vi "Calculate Vertex Array.vi"(8 "error in (no error)":errorcluster, 9 "Coordinates System":enum16{"Cartesian", "Cylindrical", "Spherical"}(ring)=enum."Spherical", 10 "3D Mesh Datatype.lvclass in":refnum<class "3D Ribbon Datatype.lvclass">, 11 "Plot Representation In":T1) -> (0 "error out":errorcluster, 1 "Dup Coordinates System":enum16{"Cartesian", "Cylindrical", "Spherical"}(ring)=enum."Spherical", 2 "3D Mesh Datatype.lvclass out":refnum<class "3D Ribbon Datatype.lvclass">, 3 "Plot Representation Out":T1)   [LabVIEW 2020, in "3D Ribbon Datatype.lvclass"]
uses:
  <vilib>/Math Plots/3D Math Plots/3D Ribbon/3D Ribbon Datatype/3D Ribbon Datatype.lvclass
  <vilib>/Math Plots/3D Math Plots/3D Plot/3D Plot/Typedef/Plot Representation.ctl
  <vilib>/Math Plots/3D Math Plots/3D Plot/3D Plot/Typedef/Range Clusters.ctl
  <vilib>/Math Plots/3D Math Plots/3D Plot/3D Plot/Typedef/Mesh Data.ctl
  <vilib>/Math Plots/3D Math Plots/3D Ribbon/3D Ribbon Datatype/3D Ribbon Datatype.lvclass/3D Ribbon Datatype.ctl
  <vilib>/Math Plots/3D Math Plots/3D Plot/3D Plot Datatype/3D Plot Datatype.lvclass
  <vilib>/Math Plots/3D Math Plots/3D Plot/3D Plot/3D Plot.lvclass
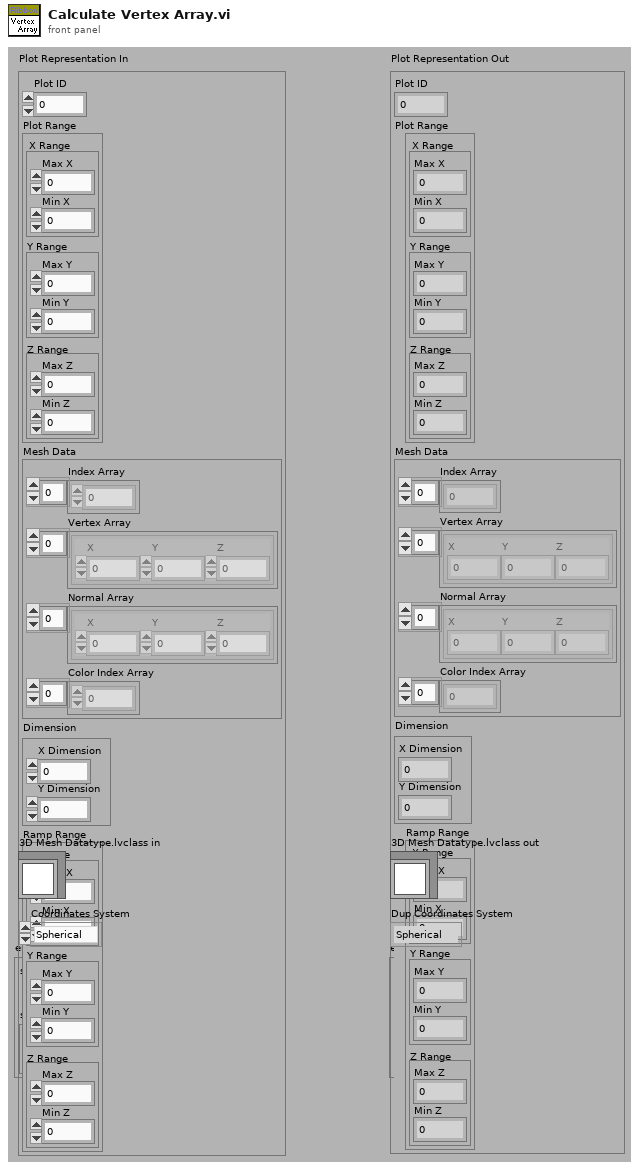
[diagram p1: front panel]
types:
  T1 = typedef "3D Plot.lvclass/Plot Representation.ctl" = cluster{"Plot ID":i32, "Plot Range":T2, "Mesh Data":T3, "Dimension":cluster{"X Dimension":i32, "Y Dimension":i32}, "Ramp Range":T2}
  T2 = typedef "3D Plot.lvclass/Range Clusters.ctl" = cluster{"X Range":cluster{"Max X":sgl, "Min X":sgl}, "Y Range":cluster{"Max Y":sgl, "Min Y":sgl}, "Z Range":cluster{"Max Z":sgl, "Min Z":sgl}}
  T3 = typedef "3D Plot.lvclass/Mesh Data.ctl" = cluster{"Index Array":u32[], "Vertex Array":cluster{"X":sgl, "Y":sgl, "Z":sgl}[], "Normal Array":cluster{"X":sgl, "Y":sgl, "Z":sgl}[], "Color Index Array":i32[]}
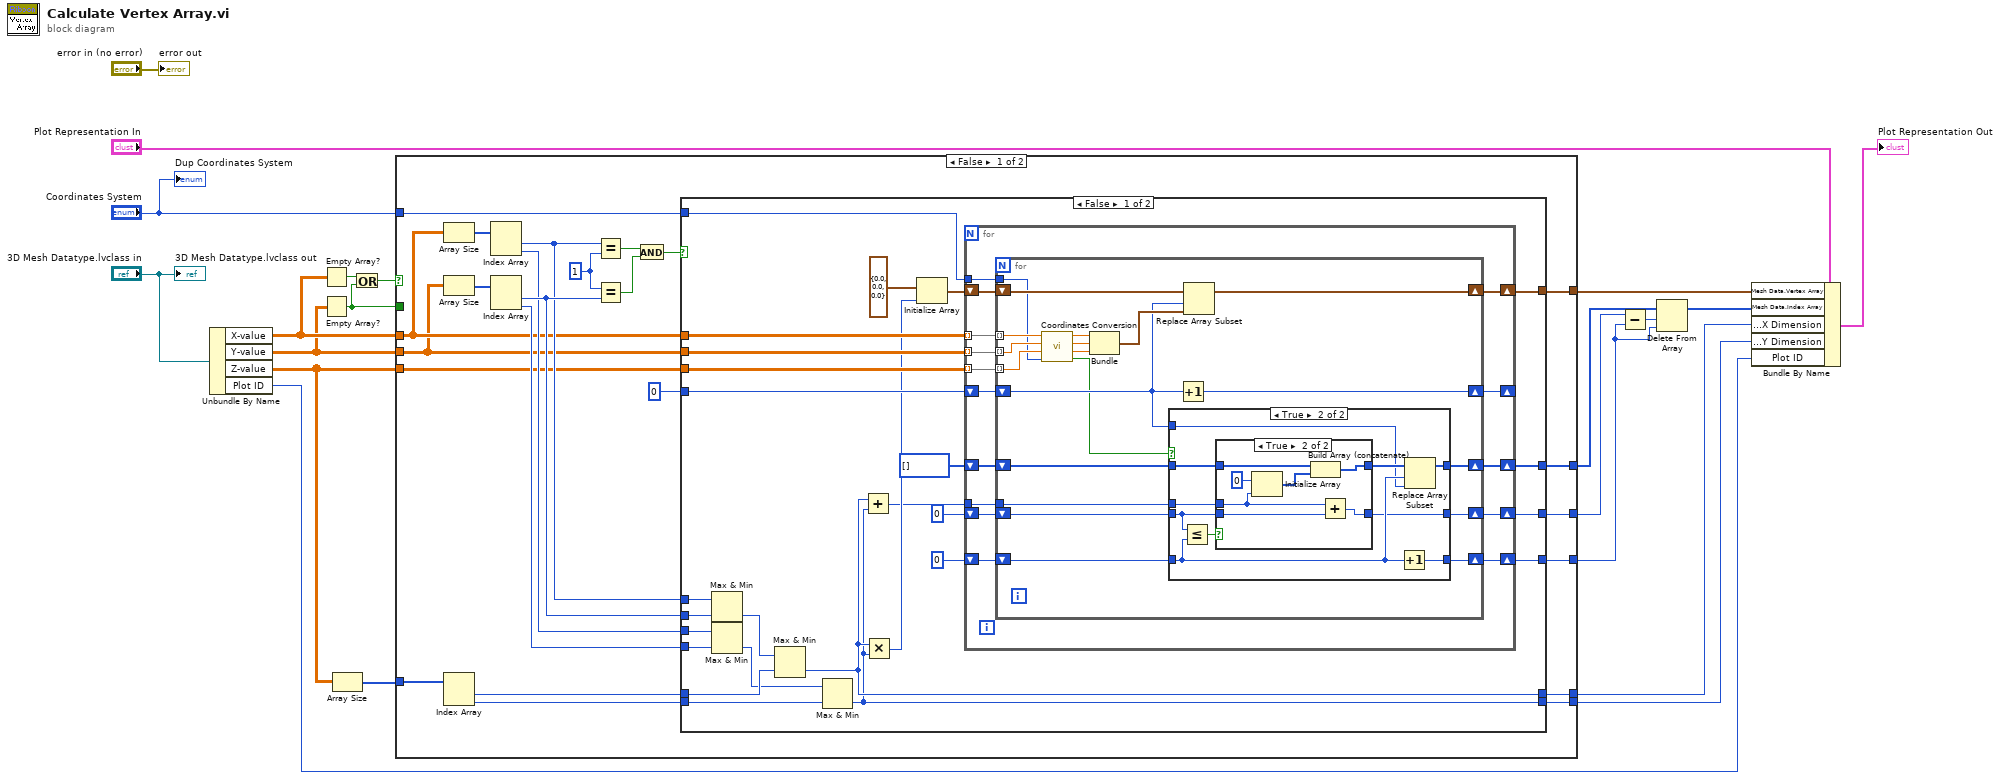
[diagram p0: block diagram]
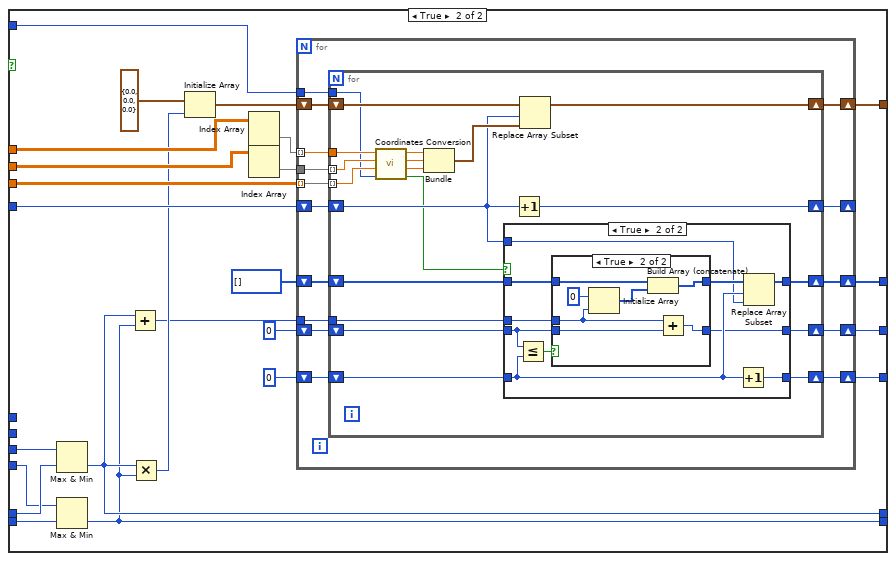
[diagram p4: hidden frame]
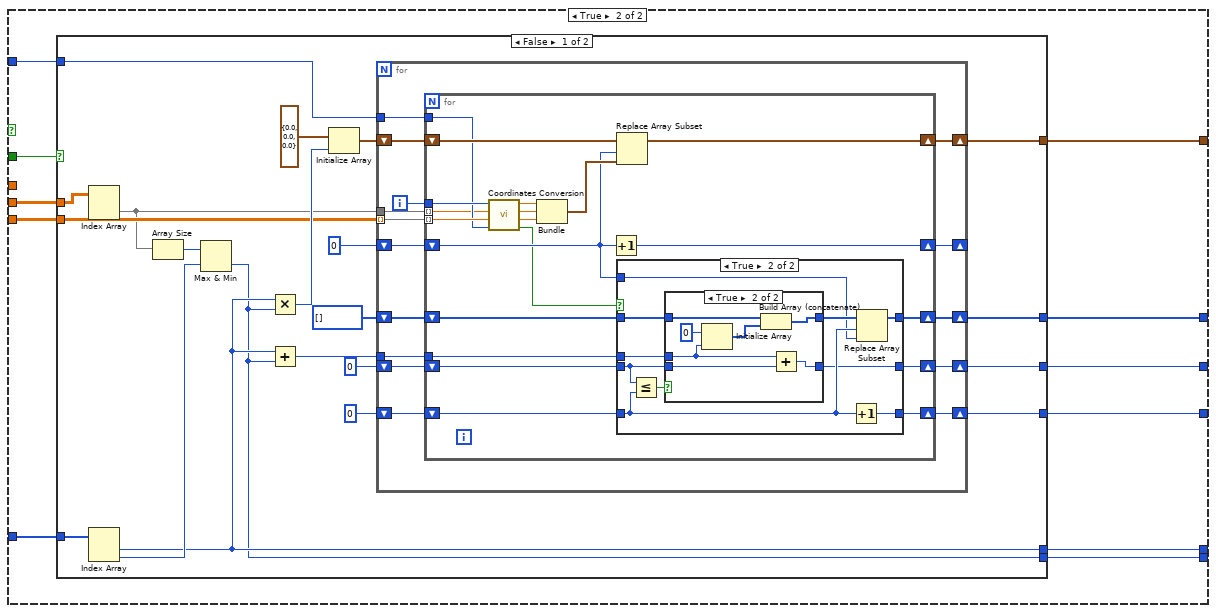
[diagram p7: hidden frame]
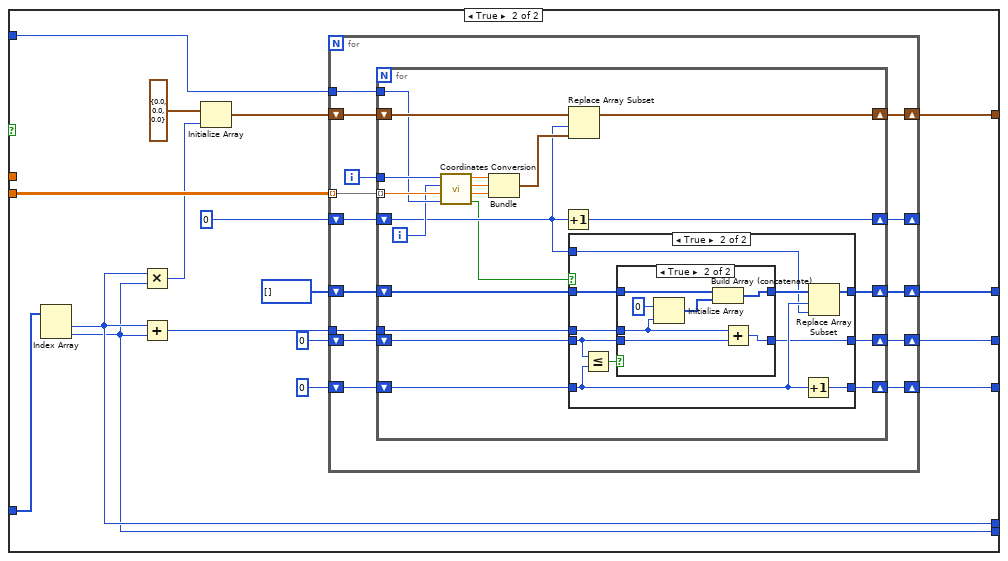
[diagram p10: hidden frame]
diagram:
  n1 = Unbundle By Name("3D Mesh Datatype.lvclass in") -> ("X-value"=w15:sgl[][], "Y-value"=w14:sgl[][], "Z-value"=w13:sgl[][], "Plot ID"=w9:i32)
  n2 = Empty Array?(array=w15) -> (empty?=w7:bool)
  n3 = Empty Array?(array=w14) -> (empty?=w6:bool)
  n4 = Array Size(array=w13) -> (size(s)=w17:i32[])
  n5 = Or(x=w7, y=w6) -> (x .or. y?=w16:bool)
  n6 = case shown="False" w16 {
    tunnel: [w25 w220] -> w12
    tunnel: w17 -> [w28 w219]
    tunnel: w13 -> [w29 w218]
    tunnel: "Coordinates System" -> [w32 w217]
    tunnel: [w27 w216] -> w11
    tunnel: [w26 w215] -> w10
    tunnel: w15 -> [w31 _]
    tunnel: w14 -> [w30 w213]
    tunnel: w6 -> [_ w214]
    tunnel: [w24 w212] -> w4
    tunnel: [w22 w211] -> w3
    tunnel: [w23 w210] -> w2
    frame False {
      w35 = 1 ("x")
      n7 = Array Size(array=w31) -> (size(s)=w33:i32[])
      n8 = Array Size(array=w30) -> (size(s)=w34:i32[])
      n9 = Index Array(array=w28) -> (element #1=w41:i32, element #2=w43:i32)  [unwired: 2 in]
      n10 = Index Array(array=w33) -> (element #1=w44:i32, element #2=w40:i32)  [unwired: 2 in]
      n11 = Index Array(array=w34) -> (element #1=w45:i32, element #2=w42:i32)  [unwired: 2 in]
      n12 = Equal?(x=w44, y=w35) -> (x = y?=w36:bool)
      n13 = Equal?(x=w35, y=w45) -> (x = y?=w37:bool)
      n14 = And(x=w36, y=w37) -> (x .and. y?=w38:bool)
      n15 = case shown="False" w38 {
        tunnel: w32 -> [w71 w152]
        tunnel: w31 -> [w70 w148]
        tunnel: w30 -> [w69 w147]
        tunnel: w29 -> [w68 w149]
        tunnel: 0 -> [w67 w150]
        tunnel: [w66 w151] -> w25
        tunnel: w40 -> [w61 w142]
        tunnel: w41 -> [w58 w141]
        tunnel: w42 -> [w60 w140]
        tunnel: w43 -> [w56 w139]
        tunnel: [w51 w134] -> w27
        tunnel: [w50 w133] -> w26
        tunnel: w44 -> [w63 _]
        tunnel: w45 -> [w62 _]
        tunnel: [w46 w131] -> w24
        tunnel: [w47 w130] -> w23
        tunnel: [w48 w129] -> w22
        frame False {
          n16 = Max & Min(x=w63, y=w62) -> (min(x,y)=w59:i32)  [unwired: 1 out]
          n17 = Max & Min(x=w61, y=w60) -> (min(x,y)=w57:i32)  [unwired: 1 out]
          n18 = Max & Min(x=w59, y=w58) -> (min(x,y)=w51:i32)  [unwired: 1 out]
          n19 = Max & Min(x=w57, y=w56) -> (min(x,y)=w50:i32)  [unwired: 1 out]
          n20 = Add(x=w51, y=w50) -> (x+y=w49:i32)
          n21 = Multiply(x=w51, y=w50) -> (x*y=w55:i32)
          n22 = Initialize Array(cluster{"X":sgl, "Y":sgl, "Z":sgl} {"X"=0.0, "Y"=0.0, "Z"=0.0} ("3D Point"), w55) -> (w64:cluster{"X":sgl, "Y":sgl, "Z":sgl}[])
          n23 = for {
            shift-right: [w85] -> w66
            shift-left: w64 -> [w86]
            tunnel: w68 -> [w84] mode=indexing
            tunnel: w70 -> [w82] mode=indexing
            tunnel: w69 -> [w83] mode=indexing
            tunnel: w71 -> [w81]
            shift-right: [w79] -> _
            shift-left: w67 -> [w80]
            shift-right: [w78] -> w46
            shift-left: u32[] [] -> [w73]
            shift-right: [w77] -> w47
            shift-left: 0 -> [w74]
            shift-right: [w76] -> w48
            shift-left: 0 -> [w75]
            tunnel: w49 -> [w72]
            n24 = for {
              tunnel: w84 -> [w102] mode=indexing
              shift-right: [w106] -> w85
              shift-left: w86 -> [w105]
              tunnel: w83 -> [w103] mode=indexing
              tunnel: w82 -> [w104] mode=indexing
              tunnel: w81 -> [w98]
              shift-right: [w96] -> w79
              shift-left: w80 -> [w95]
              shift-right: [w94] -> w78
              shift-left: w73 -> [w89]
              shift-right: [w93] -> w77
              shift-left: w74 -> [w90]
              shift-right: [w92] -> w76
              shift-left: w75 -> [w91]
              tunnel: w72 -> [w87]
              n25 = call <vilib>:"Coordinates Conversion.vi"("Coordinates System"=w98, "Z in"=w102, "Y in"=w103, "X in"=w104) -> ("NaN?"=w88:bool, "Z out"=w99:sgl, "Y out"=w100:sgl, "X out"=w101:sgl)  [unwired: 4 out]
              n26 = Bundle("X out"=w101, "Y out"=w100, "Z out"=w99) -> (w97:cluster{"X out":sgl, "Y out":sgl, "Z out":sgl})  [unwired: 1 out]
              n27 = case shown="True" w88 {
                tunnel: w89 -> [w109 w117]
                tunnel: [w109 w113] -> w94
                tunnel: w95 -> [_ w114]
                tunnel: w91 -> [w108 w115]
                tunnel: [w108 w119] -> w92
                tunnel: w90 -> [w107 w111]
                tunnel: [w107 w112] -> w93
                tunnel: w87 -> [_ w110]
                frame False {
                }
                frame True {
                  n28 = Less Or Equal?(x=w111, y=w115) -> (x <= y?=w118:bool)
                  n29 = case shown="True" w118 {
                    tunnel: w117 -> [w121 w128]
                    tunnel: [w121 w127] -> w116
                    tunnel: [w120 w123] -> w112
                    tunnel: w111 -> [w120 w124]
                    tunnel: w110 -> [_ w122]
                    frame False {
                    }
                    frame True {
                      n30 = Initialize Array(u32 0, w122) -> (w125:u32[])
                      n31 = Build Array (concatenate)(w128, w125) -> (w127:u32[])
                      n32 = Add(x=w122, y=w124) -> (x+y=w123:i32)
                    }
                  }
                  n33 = Increment(x=w115) -> (x+1=w119:i32)
                  n34 = Replace Array Subset(array=w116, new element=w114, index=w115) -> (w113:u32[])
                }
              }
              n35 = Increment(x=w95) -> (x+1=w96:i32)
              n36 = Replace Array Subset(array=w105, new element=w97, index=w95) -> (w106:cluster{"X":sgl, "Y":sgl, "Z":sgl}[])
            }
          }
        }
        frame True {
          n37 = Max & Min(x=w142, y=w141) -> (min(x,y)=w134:i32)  [unwired: 1 out]
          n38 = Max & Min(x=w140, y=w139) -> (min(x,y)=w133:i32)  [unwired: 1 out]
          n39 = Add(x=w134, y=w133) -> (x+y=w132:i32)
          n40 = Multiply(x=w134, y=w133) -> (x*y=w138:i32)
          n41 = Initialize Array(cluster{"X":sgl, "Y":sgl, "Z":sgl} {"X"=0.0, "Y"=0.0, "Z"=0.0} ("3D Point"), w138) -> (w143:cluster{"X":sgl, "Y":sgl, "Z":sgl}[])
          n42 = Index Array(array=w148) -> (element=w145:sgl[])  [unwired: 2 in]
          n43 = Index Array(array=w147) -> (element=w146:sgl[])  [unwired: 2 in]
          n44 = for {
            shift-right: [w166] -> w151
            shift-left: w143 -> [w167]
            tunnel: w149 -> [w165] mode=indexing
            tunnel: w145 -> [w163] mode=indexing
            tunnel: w146 -> [w164]
            tunnel: w152 -> [w162]
            shift-right: [w160] -> _
            shift-left: w150 -> [w161]
            shift-right: [w159] -> w131
            shift-left: u32[] [] -> [w156]
            shift-right: [w158] -> w130
            shift-left: 0 -> [w155]
            shift-right: [w157] -> w129
            shift-left: 0 -> [w154]
            tunnel: w132 -> [w153]
            n45 = for {
              tunnel: w165 -> [w183] mode=indexing
              shift-right: [w187] -> w166
              shift-left: w167 -> [w186]
              tunnel: w164 -> [w184] mode=indexing
              tunnel: w163 -> [w185]
              tunnel: w162 -> [w179]
              shift-right: [w177] -> w160
              shift-left: w161 -> [w176]
              shift-right: [w174] -> w159
              shift-left: w156 -> [w171]
              shift-right: [w173] -> w158
              shift-left: w155 -> [w169]
              shift-right: [w172] -> w157
              shift-left: w154 -> [w170]
              tunnel: w153 -> [w168]
              n46 = call <vilib>:"Coordinates Conversion.vi"("Coordinates System"=w179, "Z in"=w183, "Y in"=w184, "X in"=w185) -> ("NaN?"=w175:bool, "Z out"=w180:sgl, "Y out"=w181:sgl, "X out"=w182:sgl)  [unwired: 4 out]
              n47 = Bundle("X out"=w182, "Y out"=w181, "Z out"=w180) -> (w178:cluster{"X out":sgl, "Y out":sgl, "Z out":sgl})  [unwired: 1 out]
              n48 = case shown="True" w175 {
                tunnel: w171 -> [w190 w198]
                tunnel: [w190 w194] -> w174
                tunnel: w176 -> [_ w195]
                tunnel: w170 -> [w189 w196]
                tunnel: [w189 w200] -> w172
                tunnel: w169 -> [w188 w192]
                tunnel: [w188 w193] -> w173
                tunnel: w168 -> [_ w191]
                frame False {
                }
                frame True {
                  n49 = Less Or Equal?(x=w192, y=w196) -> (x <= y?=w199:bool)
                  n50 = case shown="True" w199 {
                    tunnel: w198 -> [w202 w209]
                    tunnel: [w202 w208] -> w197
                    tunnel: [w201 w204] -> w193
                    tunnel: w192 -> [w201 w205]
                    tunnel: w191 -> [_ w203]
                    frame False {
                    }
                    frame True {
                      n51 = Initialize Array(u32 0, w203) -> (w206:u32[])
                      n52 = Build Array (concatenate)(w209, w206) -> (w208:u32[])
                      n53 = Add(x=w203, y=w205) -> (x+y=w204:i32)
                    }
                  }
                  n54 = Increment(x=w196) -> (x+1=w200:i32)
                  n55 = Replace Array Subset(array=w197, new element=w195, index=w196) -> (w194:u32[])
                }
              }
              n56 = Increment(x=w176) -> (x+1=w177:i32)
              n57 = Replace Array Subset(array=w186, new element=w178, index=w176) -> (w187:cluster{"X":sgl, "Y":sgl, "Z":sgl}[])
            }
          }
        }
      }
    }
    frame True {
      n58 = case shown="False" w214 {
        tunnel: [w237 w315] -> w220
        tunnel: w219 -> [w236 w314]
        tunnel: w218 -> [w234 w313]
        tunnel: w217 -> [w233 w312]
        tunnel: [w226 w304] -> w216
        tunnel: [w225 w303] -> w215
        tunnel: w213 -> [w235 _]
        tunnel: [w223 w301] -> w212
        tunnel: [w221 w300] -> w211
        tunnel: [w222 w299] -> w210
        frame False {
          n59 = Index Array(array=w235) -> (element=w232:sgl[])  [unwired: 2 in]
          n60 = Index Array(array=w236) -> (element #1=w226:i32, element #2=w230:i32)  [unwired: 2 in]
          n61 = Array Size(array=w232) -> (size(s)=w231:i32)
          n62 = Max & Min(x=w231, y=w230) -> (min(x,y)=w225:i32)  [unwired: 1 out]
          n63 = Multiply(x=w226, y=w225) -> (x*y=w239:i32)
          n64 = Add(x=w226, y=w225) -> (x+y=w224:i32)
          n65 = Initialize Array(cluster{"X":sgl, "Y":sgl, "Z":sgl} {"X"=0.0, "Y"=0.0, "Z"=0.0} ("3D Point"), w239) -> (w240:cluster{"X":sgl, "Y":sgl, "Z":sgl}[])
          n66 = for {
            shift-right: [w255] -> w237
            shift-left: w240 -> [w256]
            tunnel: w234 -> [w254] mode=indexing
            tunnel: w233 -> [w253]
            shift-right: [w251] -> _
            shift-left: 0 -> [w252]
            tunnel: w232 -> [w249]
            shift-right: [w248] -> w223
            shift-left: u32[] [] -> [w243]
            shift-right: [w247] -> w222
            shift-left: 0 -> [w244]
            shift-right: [w246] -> w221
            shift-left: 0 -> [w245]
            tunnel: w224 -> [w242]
            i -> [w250]
            n67 = for {
              tunnel: w254 -> [w273] mode=indexing
              shift-right: [w276] -> w255
              shift-left: w256 -> [w275]
              tunnel: w250 -> [w274]
              tunnel: w253 -> [w269]
              shift-right: [w267] -> w251
              shift-left: w252 -> [w265]
              tunnel: w249 -> [w266] mode=indexing
              shift-right: [w263] -> w248
              shift-left: w243 -> [w258]
              shift-right: [w262] -> w247
              shift-left: w244 -> [w259]
              shift-right: [w261] -> w246
              shift-left: w245 -> [w260]
              tunnel: w242 -> [w257]
              n68 = call <vilib>:"Coordinates Conversion.vi"("Coordinates System"=w269, "Z in"=w273, "Y in"=w266, "X in"=w274) -> ("NaN?"=w264:bool, "Z out"=w270:sgl, "Y out"=w271:sgl, "X out"=w272:sgl)  [unwired: 4 out]
              n69 = Bundle("X out"=w272, "Y out"=w271, "Z out"=w270) -> (w268:cluster{"X out":sgl, "Y out":sgl, "Z out":sgl})  [unwired: 1 out]
              n70 = Increment(x=w265) -> (x+1=w267:i32)
              n71 = Replace Array Subset(array=w275, new element=w268, index=w265) -> (w276:cluster{"X":sgl, "Y":sgl, "Z":sgl}[])
              n72 = case shown="True" w264 {
                tunnel: w258 -> [w279 w287]
                tunnel: [w279 w283] -> w263
                tunnel: w265 -> [_ w284]
                tunnel: w260 -> [w278 w285]
                tunnel: [w278 w289] -> w261
                tunnel: w259 -> [w277 w281]
                tunnel: [w277 w282] -> w262
                tunnel: w257 -> [_ w280]
                frame False {
                }
                frame True {
                  n73 = Less Or Equal?(x=w281, y=w285) -> (x <= y?=w288:bool)
                  n74 = case shown="True" w288 {
                    tunnel: w287 -> [w291 w298]
                    tunnel: [w291 w297] -> w286
                    tunnel: [w290 w293] -> w282
                    tunnel: w281 -> [w290 w294]
                    tunnel: w280 -> [_ w292]
                    frame False {
                    }
                    frame True {
                      n75 = Initialize Array(u32 0, w292) -> (w295:u32[])
                      n76 = Build Array (concatenate)(w298, w295) -> (w297:u32[])
                      n77 = Add(x=w292, y=w294) -> (x+y=w293:i32)
                    }
                  }
                  n78 = Increment(x=w285) -> (x+1=w289:i32)
                  n79 = Replace Array Subset(array=w286, new element=w284, index=w285) -> (w283:u32[])
                }
              }
            }
          }
        }
        frame True {
          n80 = Index Array(array=w314) -> (element #1=w304:i32, element #2=w303:i32)  [unwired: 2 in]
          n81 = Multiply(x=w304, y=w303) -> (x*y=w309:i32)
          n82 = Add(x=w304, y=w303) -> (x+y=w302:i32)
          n83 = Initialize Array(cluster{"X":sgl, "Y":sgl, "Z":sgl} {"X"=0.0, "Y"=0.0, "Z"=0.0} ("3D Point"), w309) -> (w310:cluster{"X":sgl, "Y":sgl, "Z":sgl}[])
          n84 = for {
            shift-right: [w328] -> w315
            shift-left: w310 -> [w329]
            tunnel: w313 -> [w327] mode=indexing
            tunnel: w312 -> [w326]
            shift-right: [w324] -> _
            shift-left: 0 -> [w325]
            shift-right: [w320] -> w300
            shift-left: 0 -> [w317]
            shift-right: [w321] -> w299
            shift-left: 0 -> [w318]
            shift-right: [w322] -> w301
            shift-left: u32[] [] -> [w319]
            tunnel: w302 -> [w316]
            i -> [w323]
            n85 = for {
              tunnel: w327 -> [w346] mode=indexing
              shift-right: [w349] -> w328
              shift-left: w329 -> [w348]
              tunnel: w323 -> [w347]
              tunnel: w326 -> [w342]
              shift-right: [w340] -> w324
              shift-left: w325 -> [w334]
              shift-right: [w338] -> w322
              shift-left: w319 -> [w335]
              shift-right: [w337] -> w321
              shift-left: w318 -> [w331]
              shift-right: [w336] -> w320
              shift-left: w317 -> [w332]
              tunnel: w316 -> [w330]
              i -> [w339]
              n86 = call <vilib>:"Coordinates Conversion.vi"("Coordinates System"=w342, "Z in"=w346, "Y in"=w339, "X in"=w347) -> ("NaN?"=w333:bool, "Z out"=w343:sgl, "Y out"=w344:sgl, "X out"=w345:sgl)  [unwired: 4 out]
              n87 = Bundle("X out"=w345, "Y out"=w344, "Z out"=w343) -> (w341:cluster{"X out":sgl, "Y out":sgl, "Z out":sgl})  [unwired: 1 out]
              n88 = Increment(x=w334) -> (x+1=w340:i32)
              n89 = Replace Array Subset(array=w348, new element=w341, index=w334) -> (w349:cluster{"X":sgl, "Y":sgl, "Z":sgl}[])
              n90 = case shown="True" w333 {
                tunnel: w335 -> [w352 w360]
                tunnel: [w352 w356] -> w338
                tunnel: w334 -> [_ w357]
                tunnel: w332 -> [w351 w358]
                tunnel: [w351 w362] -> w336
                tunnel: w331 -> [w350 w354]
                tunnel: [w350 w355] -> w337
                tunnel: w330 -> [_ w353]
                frame False {
                }
                frame True {
                  n91 = Less Or Equal?(x=w354, y=w358) -> (x <= y?=w361:bool)
                  n92 = case shown="True" w361 {
                    tunnel: w360 -> [w364 w371]
                    tunnel: [w364 w370] -> w359
                    tunnel: [w363 w366] -> w355
                    tunnel: w354 -> [w363 w367]
                    tunnel: w353 -> [_ w365]
                    frame False {
                    }
                    frame True {
                      n93 = Initialize Array(u32 0, w365) -> (w368:u32[])
                      n94 = Build Array (concatenate)(w371, w368) -> (w370:u32[])
                      n95 = Add(x=w365, y=w367) -> (x+y=w366:i32)
                    }
                  }
                  n96 = Increment(x=w358) -> (x+1=w362:i32)
                  n97 = Replace Array Subset(array=w359, new element=w357, index=w358) -> (w356:u32[])
                }
              }
            }
          }
        }
      }
    }
  }
  n98 = Subtract(x=w2, y=w3) -> (x-y=w5:i32)
  n99 = Delete From Array(array=w4, length=w5, index=w3) -> (array with subset deleted=w1:u32[])  [unwired: 1 out]
  n100 = Bundle By Name(cluster="Plot Representation In", "Mesh Data.Vertex Array"=w12, "Mesh Data.Index Array"=w1, "Dimension.X Dimension"=w11, "Dimension.Y Dimension"=w10, "Plot ID"=w9) -> (→"Plot Representation Out":T1)
  "error out" <- "error in (no error)"
  "3D Mesh Datatype.lvclass out" <- "3D Mesh Datatype.lvclass in"
  "Dup Coordinates System" <- "Coordinates System"
